vi "HFRR ADV v10.vi"() -> ()   [LabVIEW 2025] (continued)
            }
            "Rt 3" <- TRUE ("Rt 3")
          }
        }
        n2649 = case shown="True" w3152 {
          tunnel: [FALSE ("RUN") TRUE ("RUN")] -> w3151
          tunnel: [_ 2] -> w3145
          frame False {
          }
          frame True {
          }
        }
        n2650 = case shown="True" w3150 {
          tunnel: [FALSE ("RUN") TRUE ("RUN")] -> w3149
          tunnel: [_ 3] -> w3144
          frame False {
          }
          frame True {
          }
        }
        n2651 = case shown="\"Acquire\"" w3130 {
          tunnel: w3132 -> [_ w3363]
          frame Default {
            w3362 = 0.0 ("output")
            n2652 = local write "PID-out"(w3362) -> ()
            n2653 = local write "Frequency ( Hz )"(w3362) -> ()
          }
          frame "Acquire" {
            n2654 = stacked-sequence {
              frame #0 {
                n2655 = local read "Auto Start Test"() -> (w3365:bool)
                n2656 = case shown="True" w3365 {
                  tunnel: "RUN" -> [w3386 w3389]
                  tunnel: [w3386 w3388] -> w3366
                  frame False {
                  }
                  frame True {
                    n2657 = local read "Auto Start Temp"() -> (w3387:bool)
                    n2658 = Or(x=w3389, y=w3387) -> (x .or. y?=w3388:bool)
                  }
                }
                n2659 = local read "clk"() -> (w3385:dbl)
                n2660 = local read "Save"() -> (w3381:bool)
                n2661 = Equal?(x=w3385, y=0.0) -> (x = y?=w3382:bool)
                n2662 = And(x=w3382, y=w3381) -> (x .and. y?=w3383:bool)
                n2663 = Not(x="Engage") -> (.not. x?=w3372:bool)
                n2664 = case shown="True" w3366 {
                  tunnel: [w3397 w3415] -> w3368
                  frame False {
                    w3397 = 0.0
                    n2665 = local read "Auto Start Test"() -> (w3393:bool)
                    n2666 = local write "Reinit PID"(TRUE) -> ()
                    n2667 = local write "Start Time"(TRUE ("Start Time")) -> ()
                    n2668 = property on="Stroke" class="DigNum (strict)"("Visible"=TRUE) -> ()  [unwired: 2 in, 2 out]
                    n2669 = property on="Stroke 2" class="DigNum (strict)"("Visible"=FALSE) -> ()  [unwired: 2 in, 2 out]
                    n2670 = case shown="False" w3393 {
                      frame False {
                        n2671 = property on="Heater Button" class="Bool (strict)"("DisabledEnum"=T16."Enabled" ("Disabled")) -> ()  [unwired: 2 in, 2 out]
                        n2672 = property on="Humidity" class="Bool (strict)"("DisabledEnum"=T16."Enabled" ("Disabled")) -> ()  [unwired: 2 in, 2 out]
                      }
                      frame True {
                      }
                    }
                    n2673 = case shown="False" "TestCompFlg" {
                      frame False {
                        n2674 = local read "StartFlg"() -> (w3403:bool)
                        n2675 = case shown="True" w3403 {
                          frame False {
                          }
                          frame True {
                            n2676 = flat-sequence {
                              frame #0 {
                                n2677 = local read "EVENT LOG"() -> (w3405:string)
                                n2678 = call "Event Log.vi"("Content"="Test was interrupted", "EVENT LOG"=w3405) -> ("EVENT LOG"=w3406:string)  [unwired: 8 in, 1 out]
                                n2679 = local write "EVENT LOG"(w3406) -> ()
                              }
                              frame #1 {
                                w3407 = FALSE ("StartFlg")
                                n2680 = local write "Heater Button"(w3407) -> ()
                                n2681 = local write "StartFlg"(w3407) -> ()
                                n2682 = local write "Humidity"(w3407) -> ()
                              }
                            }
                          }
                        }
                      }
                      frame True {
                      }
                    }
                    n2683 = local write "String 14"("Test will autostart once parameters reach the set value." ("String 14")) -> ()
                    n2684 = local write "Old Pid Val"(w3397) -> ()
                  }
                  frame True {
                    n2685 = property on="Stroke 2" class="DigNum (strict)"("Visible"=TRUE) -> ()  [unwired: 2 in, 2 out]
                    n2686 = property on="Stroke" class="DigNum (strict)"("Visible"=FALSE) -> ()  [unwired: 2 in, 2 out]
                    n2687 = property on="STOP 2" class="Bool (strict)"("Disabled"=u8 2) -> ()  [unwired: 2 in, 2 out]
                    n2688 = local write "String 14"(" Running....." ("String 14")) -> ()
                    n2689 = property on="Heater Button" class="Bool (strict)"("DisabledEnum"=T16."Disabled and Grayed Out" ("Disabled")) -> ()  [unwired: 2 in, 2 out]
                    n2690 = property on="Humidity" class="Bool (strict)"("DisabledEnum"=T16."Disabled and Grayed Out" ("Disabled")) -> ()  [unwired: 2 in, 2 out]
                    n2691 = local read "PID Ref"() -> (w3426:bool)
                    n2692 = case shown="True" w3426 {
                      tunnel: [w3432 w3448] -> w3425
                      frame False {
                        n2693 = local read "Old Pid Val"() -> (w3432:dbl)
                      }
                      frame True {
                        n2694 = local read "Set Hz"() -> (w3441:dbl)
                        n2695 = local read "Frequency"() -> (w3452:dbl)
                        n2696 = Add(x=w3441, y=10.0) -> (x+y=w3450:dbl)
                        n2697 = Add(x=w3441, y=-10.0 ("Offset")) -> (x+y=w3459:dbl)
                        n2698 = Add(x=w3441, y=-10.0) -> (x+y=w3451:dbl)
                        n2699 = In Range and Coerce(upper limit=w3450, x=w3452, lower limit=w3451) -> (coerced(x)=w3440:dbl)  [unwired: 1 out]
                        n2700 = Or(x="Reinit PID", y="Reinit PID") -> (x .or. y?=w3449:bool)
                        n2701 = Multiply(x=w3459, y=0.1 ("Gain")) -> (x*y=w3438:dbl)
                        n2702 = local read "Elapsed time"() -> (w3445:dbl)
                        n2703 = local read "SPEED OUT:"() -> (w3460:dbl)
                        n2704 = Add(x=w3438, y=1.5) -> (x+y=w3436:dbl)
                        n2705 = call-poly <vilib>:"PID.vi"("reinitialize? (F)"=w3449, "output range"=cluster{"output high":dbl, "output low":dbl} {"output high"=1.0, "output low"=-1.0}, "PID gains"=T13 {"proportional gain (Kc)"=0.0005, "integral time (Ti, min)"=0.001, "derivative time (Td, min)"=0.0} ("Motor PID"), "process variable"=w3440, "setpoint"=w3441) -> ("output"=w3439:dbl)  [unwired: 5 in, 1 out]
                        n2706 = Multiply(x=w3436, y=w3460) -> (x*y=w3435:dbl)
                        n2707 = Greater?(x=w3445, y=0.05) -> (0:w3444:bool)
                        n2708 = case shown="True" w3444 {
                          tunnel: w3439 -> [_ w3462]
                          tunnel: [0.0 ("output") w3462] -> w3442
                          frame False {
                          }
                          frame True {
                            n2709 = local write "Reinit PID"(FALSE ("Reinit PID")) -> ()
                          }
                        }
                        n2710 = Multiply(x=w3435, y=0.8) -> (x*y=w3434:dbl)
                        n2711 = Add(x=w3434, y=w3442) -> (x+y=w3447:dbl)
                        n2712 = flat-sequence {
                          tunnel: [w3465] -> w3448
                          tunnel: w3447 -> [w3465]
                          frame #0 {
                            n2713 = local write "PID Ref"(FALSE ("PID Ref")) -> ()
                          }
                        }
                      }
                    }
                    "Old Pid Val" <- w3425
                    n2714 = case shown="True" "Start Time" {
                      selector: "Start Time" -> [_ w3428]
                      frame False {
                      }
                      frame True {
                        n2715 = Not(x=w3428) -> (.not. x?=w3427:bool)
                        n2716 = local write "Start Time"(w3427) -> ()
                        n2717 = local read "EVENT LOG"() -> (w3429:string)
                        n2718 = call "Event Log.vi"("Content"="Test in progress", "EVENT LOG"=w3429) -> ("EVENT LOG"=w3431:string)  [unwired: 8 in, 1 out]
                        n2719 = local write "EVENT LOG"(w3431) -> ()
                      }
                    }
                    n2720 = local read "Set Hz"() -> (w3422:dbl)
                    n2721 = call <vilib>:"Uniform White Noise Waveform.vi"() -> ("signal out"=w3421:waveform(dbl))  [unwired: 10 in, 1 out]
                    n2722 = local read "Freq"() -> (w3414:dbl)
                    n2723 = Add(x=w3422, y=w3421) -> (x+y=w3420:waveform(dbl))
                    n2724 = Multiply(x=w3420, y=ext 0.1) -> (x*y=w3416:waveform(ext))
                    n2725 = Multiply(x=w3414, y=0.9) -> (x*y=w3417:dbl)
                    n2726 = Add(x=w3416, y=w3417) -> (x+y=w3415:waveform(ext))
                    "StartFlg" <- TRUE ("StartFlg")
                  }
                }
                n2727 = case shown="True" w3383 {
                  frame False {
                  }
                  frame True {
                    n2728 = local write "clk"(10.0 ("clk")) -> ()
                    n2729 = Get Date/Time In Seconds() -> (seconds since 1Jan1904=w3468:timestamp)
                    n2730 = To Double Precision Float(number=w3468) -> (double precision float=w3466:dbl)
                    n2731 = local write "acq timer"(w3466) -> ()
                    n2732 = local write "act save time"(w3466) -> ()
                  }
                }
                n2733 = call "Elapsed Time"("Time Target (s)"="Countdown", "Reset"=w3372) -> ("Elapsed Time (s)"=w3377:dbl, "Time has Elapsed"=w3375:bool)  [unwired: 10 in, 6 out]
                "Countdown 2" <- w3377
                n2734 = Subtract(x=w3377, y=2.0) -> (x-y=w3380:dbl)
                n2735 = Less?(x=w3380, y="Countdown") -> (x < y?=w3378:bool)
                n2736 = And(x=w3378, y=w3375) -> (x .and. y?=w3374:bool)
                n2737 = case shown="True" w3374 {
                  frame False {
                  }
                  frame True {
                    (unwired) dbl[] [] ("History Data")
                    n2738 = local write "Engage"(FALSE ("Engage")) -> ()
                    n2739 = local write "RUN"(TRUE ("RUN")) -> ()
                    n2740 = local read "Humidity ( %RH )"() -> (→"Rh Before":dbl)
                  }
                }
                n2741 = local read "Test \nStatus"() -> (w3370:bool)
                n2742 = Select(t=w3368, s=w3370, f=0.0) -> (s? t:f=w3369:dbl)
                n2743 = local write "Frequency ( Hz )"(w3369) -> ()
                n2744 = local write "Freq"(w3369) -> ()
              }
              frame #1 {
                w3491 = 1000000.0 ("x")
                # "Elapsed time\ncof\nstroke\nAir temp\nTemp\nHumidity"
                # "acq timer\n\nact save time"
                # "convert to microseconds"
                n2745 = local read "COUNT"() -> (w3474:i32)
                n2746 = local read "Rate"() -> (w3487:dbl)
                n2747 = Divide(x=w3491, y=w3487) -> (x/y=w3492:dbl)
                n2748 = Greater Or Equal?(x=w3474, y=250) -> (x >= y?=w3473:bool)
                n2749 = Get Date/Time In Seconds() -> (seconds since 1Jan1904=w3494:timestamp)
                n2750 = case shown="True" w3473 {
                  frame False {
                    n2751 = local read "COUNT"() -> (w3495:i32)
                    n2752 = Increment(x=w3495) -> (x+1=w3496:i32)
                    n2753 = local write "COUNT"(w3496) -> ()
                  }
                  frame True {
                    n2754 = local write "COUNT"(0 ("COUNT")) -> ()
                  }
                }
                n2755 = local read "Samplingtime 2"() -> (w3472:dbl)
                n2756 = local read "act save time"() -> (w3489:dbl)
                n2757 = Divide(x=w3492, y=w3491) -> (x/y=w3490:dbl)
                n2758 = To Double Precision Float(number=w3494) -> (double precision float=w3483:dbl)
                n2759 = Add(x=w3489, y=w3472) -> (x+y=w3488:dbl)
                n2760 = local read "acq timer"() -> (w3493:dbl)
                n2761 = local read "COUNT"() -> (w3476:i32)
                n2762 = Greater Or Equal?(x=w3483, y=w3488) -> (x >= y?=w3471:bool)
                n2763 = Multiply(x=w3490, y=w3476) -> (x*y=w3482:dbl)
                n2764 = Subtract(x=w3483, y=w3493) -> (x-y=w3485:dbl)
                n2765 = local read "Save"() -> (w3486:bool)
                n2766 = Add(x=w3485, y=w3482) -> (x+y=w3469:dbl)
                "Elapsed time 3" <- w3469
                n2767 = And(x=w3471, y=w3486) -> (x .and. y?=w3484:bool)
                n2768 = Divide(x=w3469, y=60.0) -> (x/y=w3480:dbl)
                n2769 = local read "Test \nStatus"() -> (w3470:bool)
                n2770 = local read "clk"() -> (w3477:dbl)
                n2771 = Equal?(x=w3477, y=10.0) -> (x = y?=w3479:bool)
                n2772 = case shown="True" w3484 {
                  tunnel: w3483 -> [_ w3598]
                  tunnel: [FALSE ("Boolean 2") TRUE ("Boolean 2")] -> _
                  frame False {
                  }
                  frame True {
                    w3545 = ";" ("Substring")
                    # "Pid out/\nFreq response value"
                    n2773 = local write "act save time"(w3598) -> ()
                    n2774 = local read "FILE"() -> (w3539:string)
                    n2775 = call "file check.vi"("file name in"=w3539) -> ("error out"=w3542:errorcluster, "file name out"=w3537:string)  [unwired: 9 in]
                    n2776 = call "FILE PATH CREATION.vi"("error in"=w3542, "FILE NAME :"=w3537) -> ("FILE OUT"=w3540:path)  [unwired: 8 in, 1 out]
                    n2777 = Concatenate Strings(w3537, ".dgf" ("Substring")) -> (w3541:string)
                    n2778 = local read "Set Strk"() -> (w3569:dbl)
                    n2779 = local read "Stroke"() -> (w3560:dbl)
                    n2780 = local read "FF 2"() -> (→"Frictional Force ( N )" →"Frictional Force ( N )":dbl)
                    n2781 = Build Path(base path=w3540, name or relative path=w3541) -> (appended path=w3536:path)
                    n2782 = Subtract(x=w3560, y=w3569) -> (x-y=w3566:dbl)
                    n2783 = local read "COF 2"() -> (w3551:dbl)
                    "cof" <- w3551
                    "Coefficient of Friction" <- w3551
                    "COF 4" <- w3551
                    "Coefficient of Friction" <- w3551
                    n2784 = Multiply(x=w3566, y=0.05) -> (x*y=w3568:dbl)
                    n2785 = local read "TEMP"() -> (w3555:dbl)
                    "Temp" <- w3555
                    "Temperature ( Deg C )" <- w3555
                    n2786 = Add(x=w3568, y=w3569) -> (x+y=w3549:dbl)
                    "Stroke Ln" <- w3549
                    "Disp" <- w3549
                    n2787 = local read "ecr"() -> (w3552:dbl)
                    "Electrical Contact Resistance ( % )" <- w3552
                    n2788 = local read "Humidity ( %RH )"() -> (w3554:dbl)
                    "Humidity ( %RH )" <- w3554
                    "Humidity ( %RH )" <- w3554
                    n2789 = local read "Frequency ( Hz )"() -> (w3562:dbl)
                    n2790 = local read "Elapsed time"() -> (w3591:dbl)
                    n2791 = disable-structure shown="Disabled" {
                      frame Disabled {
                        n2792 = local read "ecr 3"() -> ()  [unwired: 1 in]
                      }
                      frame Enabled {
                      }
                    }
                    n2793 = local read "AIR TEMP"() -> (w3559:dbl)
                    n2794 = local read "PID-out"() -> (w3565:dbl)
                    n2795 = local write "Temperature ( Deg C )"(w3555) -> ()
                    n2796 = Number To Fractional String(number=w3549, width (-)=i16 9 ("precision (6)"), precision (6)=i16 6) -> (F-format string=w3584:string)  [unwired: 1 in]
                    n2797 = Number To Fractional String(number=w3559, width (-)=i16 9 ("precision (6)"), precision (6)=i16 3) -> (F-format string=w3583:string)  [unwired: 1 in]
                    n2798 = Number To Fractional String(number=w3555, width (-)=i16 9 ("precision (6)"), precision (6)=i16 3) -> (F-format string=w3580:string)  [unwired: 1 in]
                    n2799 = Number To Fractional String(number=w3554, width (-)=i16 9 ("precision (6)"), precision (6)=i16 3) -> (F-format string=w3577:string)  [unwired: 1 in]
                    n2800 = Number To Fractional String(number=w3552, width (-)=i16 9 ("precision (6)"), precision (6)=i16 3) -> (F-format string=w3574:string)  [unwired: 1 in]
                    n2801 = Number To Fractional String(number=w3565, width (-)=i16 9 ("precision (6)"), precision (6)=i16 3) -> (F-format string=w3570:string)  [unwired: 1 in]
                    n2802 = Number To Fractional String(number=w3562, width (-)=i16 9 ("precision (6)"), precision (6)=i16 3) -> (F-format string=w3561:string)  [unwired: 1 in]
                    n2803 = Number To Fractional String(number=w3551, width (-)=i16 9 ("precision (6)"), precision (6)=i16 6) -> (F-format string=w3592:string)  [unwired: 1 in]
                    n2804 = Number To Fractional String(number=w3591, width (-)=i16 14 ("precision (6)"), precision (6)=i16 3) -> (F-format string=w3593:string)  [unwired: 1 in]
                    n2805 = Bundle("y"=1.02, w3549, "y"=0.98) -> (w3553:cluster{"y":dbl, dbl, "y":dbl})  [unwired: 1 in]
                    n2806 = Number To Fractional String(number="Ambient Humidity :", width (-)=i16 9 ("precision (6)"), precision (6)=i16 6) -> (F-format string=w3543:string)  [unwired: 1 in]
                    n2807 = local read "RUN"() -> (w3550:bool)
                    n2808 = case shown="True" w3550 {
                      tunnel: w3553 -> [_ w3603]
                      tunnel: w3549 -> [_ w3602]
                      tunnel: w3549 -> [_ w3601]
                      tunnel: w3549 -> [_ w3600]
                      frame False {
                      }
                      frame True {
                        "Stroke ( mm )" <- w3603
                        "Stroke ( mm )" <- w3603
                        "Stroke 4" <- w3602
                        "Stroke 3" <- w3601
                        "Stroke 2" <- w3600
                      }
                    }
                    n2809 = Concatenate Strings(w3593, w3545, w3592, w3545, w3584, w3545, w3583, w3545, w3580, w3545, w3577, w3545, w3574, w3545, w3570, w3545, w3561, w3545, w3543, "\r") -> (w3590:string)
                    n2810 = call <vilib>:"Write Characters To File.vi"("append to file? (new file:F)"=TRUE, "character string"=w3590, "file path (dialog if empty)"=w3536) -> ()  [unwired: 2 in, 1 out]
                    "refresh flag" <- TRUE ("refresh flag")
                  }
                }
                n2811 = case shown="True" w3470 {
                  tunnel: w3480 -> [_ w3506]
                  tunnel: w3485 -> [_ w3516]
                  tunnel: [0.0 w3512] -> _
                  tunnel: w3479 -> [_ w3511]
                  tunnel: [0.0 w3510] -> _
                  tunnel: w3469 -> [_ w3510]
                  tunnel: w3483 -> [w3499 _]
                  frame False {
                    n2812 = local write "acq timer"(w3499) -> ()
                    n2813 = local write "Test Duration Status"(0.0 ("Test Duration Status")) -> ()
                  }
                  frame True {
                    n2814 = local read "Set Hz"() -> (w3513:dbl)
                    n2815 = local write "Elapsed time"(w3506) -> ()
                    n2816 = local read "test time"() -> (w3505:dbl)
                    n2817 = Multiply(x=w3516, y=w3513) -> (x*y=w3515:dbl)
                    n2818 = case shown="False" w3511 {
                      tunnel: w3515 -> [w3517 _]
                      tunnel: [w3517 1.0] -> w3512
                      frame False {
                        n2819 = local write "Cycles elapsed"(w3517) -> ()
                      }
                      frame True {
                      }
                    }
                    n2820 = Greater?(x=w3506, y=w3505) -> (0:w3514:bool)
                    n2821 = Subtract(x=w3505, y=w3506) -> (x-y=w3504:dbl)
                    "time" <- w3504
                    n2822 = Multiply(x=w3504, y=60.0) -> (x*y=w3503:dbl)
                    n2823 = local write "Time Remaining"(w3503) -> ()
                    n2824 = local write "Remaining Time"(w3503) -> ()
                    n2825 = case shown="True" w3514 {
                      frame False {
                      }
                      frame True {
                        w3519 = T16."Enabled" ("Disabled")
                        w3523 = "" ("FILE")
                        w3524 = TRUE ("Visible")
                        n2826 = local write "Humidity"(FALSE ("Humidity")) -> ()
                        n2827 = local write "RUN"(FALSE ("OK Button 2")) -> ()
                        n2828 = local write "Heater Button"(FALSE ("Heater Button")) -> ()
                        n2829 = local write "Auto Start Test"(FALSE ("Auto Start Test")) -> ()
                        n2830 = local write "TestCompFlg"(TRUE ("StpFlg")) -> ()
                        n2831 = local read "Humidity ( %RH )"() -> (→"Rh After":dbl)
                        n2832 = property on="STOP 2" class="Bool (strict)"("Disabled"=u8 0) -> ()  [unwired: 2 in, 2 out]
                        n2833 = local read "EVENT LOG"() -> (w3529:string)
                        n2834 = call "Event Log.vi"("Content"="Test Completed", "EVENT LOG"=w3529) -> ("EVENT LOG"=w3528:string)  [unwired: 8 in, 1 out]
                        n2835 = property on="RUN" class="Bool (strict)"("Visible"=w3524) -> ()  [unwired: 2 in, 2 out]
                        n2836 = property on="Auto Start Test" class="Bool (strict)"("Visible"=w3524) -> ()  [unwired: 2 in, 2 out]
                        n2837 = local write "Batch Ref Num :"(w3523) -> ()
                        n2838 = local write "FILE"(w3523) -> ()
                        n2839 = local write "EVENT LOG"(w3528) -> ()
                        n2840 = local write "TEST FILE NAM,E SAVED"(FALSE ("TEST FILE NAM,E SAVED")) -> ()
                        n2841 = local write "Fuel Discription :"(w3523) -> ()
                        n2842 = local write "Remarks :"(w3523) -> ()
                        n2843 = local write "Main Dashboard Buttons"(T1."Imaging" ("Main Dashboard Buttons")) -> ()
                        n2844 = local write "Main Tab"(T2."Adv Scar" ("Main Tab")) -> ()
                        n2845 = property on="FRICVALZ 2" class="Bool (strict)"("DisabledEnum"=w3519) -> ()  [unwired: 2 in, 2 out]
                        n2846 = property on="FRICVALZ 3" class="Bool (strict)"("DisabledEnum"=w3519) -> ()  [unwired: 2 in, 2 out]
                        n2847 = property on="FRICVALZ 4" class="Bool (strict)"("DisabledEnum"=w3519) -> ()  [unwired: 2 in, 2 out]
                      }
                    }
                    n2848 = Divide(x=w3506, y=w3505) -> (x/y=w3509:dbl)
                    n2849 = Multiply(x=w3509, y=100.0) -> (x*y=w3507:dbl)
                    n2850 = local write "Test Duration Status"(w3507) -> ()
                  }
                }
              }
              frame #2 {
                n2851 = case shown="True" "Heater Button" {
                  tunnel: [0.0 ("output") w3627] -> w3604
                  frame False {
                    w3607 = TRUE ("tmpchk")
                    n2852 = local read "TEMP"() -> (w3608:dbl)
                    n2853 = local write "Temp ini"(w3608) -> ()
                    n2854 = local write "Reset 4"(w3607) -> ()
                    n2855 = local write "tmpchk"(w3607) -> ()
                    n2856 = local write "reinit"(TRUE ("reinit")) -> ()
                    n2857 = local write "manual temp log"(TRUE ("manual temp log")) -> ()
                  }
                  frame True {
                    # "Logic to turn off\nthe heater when \ntemp is not rising.\nTime - 60 sec\nDelta t- 5°c"
                    n2858 = local read "Temp ini"() -> (w3615:dbl)
                    n2859 = local read "Auto Start Test"() -> (w3611:bool)
                    n2860 = Less?(x=w3615, y=53.0) -> (x < y?=w3613:bool)
                    n2861 = case shown="False" w3611 {
                      frame False {
                        n2862 = local read "Set Temp"() -> (w3638:dbl)
                        n2863 = local read "TEMP"() -> (w3637:dbl)
                        n2864 = Subtract(x=w3638, y=w3637) -> (x-y=w3636:dbl)
                        n2865 = Absolute Value(x=w3636) -> (abs(x)=w3635:dbl)
                        n2866 = Less?(x=w3635, y=0.5) -> (x < y?=w3633:bool)
                        n2867 = case shown="True" w3633 {
                          tunnel: "manual temp log" -> [_ w3639]
                          frame False {
                          }
                          frame True {
                            n2868 = case shown="True" w3639 {
                              selector: w3639 -> [_ w3640]
                              frame False {
                              }
                              frame True {
                                # "#Event log"
                                n2869 = Not(x=w3640) -> (.not. x?=w3641:bool)
                                n2870 = local write "manual temp log"(w3641) -> ()
                                n2871 = local read "EVENT LOG"() -> (w3644:string)
                                n2872 = call "Event Log.vi"("Content"="Target Temperature reached", "EVENT LOG"=w3644) -> ("EVENT LOG"=w3643:string)  [unwired: 8 in, 1 out]
                                n2873 = local write "EVENT LOG"(w3643) -> ()
                              }
                            }
                          }
                        }
                      }
                      frame True {
                        n2874 = local write "manual temp log"(TRUE ("manual temp log")) -> ()
                      }
                    }
                    n2875 = And(x="tmpchk", y=w3613) -> (x .and. y?=w3616:bool)
                    n2876 = case shown="True" w3616 {
                      frame False {
                      }
                      frame True {
                        n2877 = call "Elapsed Time8"("Time Target (s)"=300.0, "Reset"="Reset 4") -> ("Time has Elapsed"=w3646:bool)  [unwired: 10 in, 7 out]
                        n2878 = flat-sequence {
                          tunnel: w3646 -> [_]
                          frame #0 {
                            n2879 = local write "Reset 4"(FALSE ("Reset 4")) -> ()
                          }
                        }
                        n2880 = case shown="True" w3646 {
                          frame False {
                          }
                          frame True {
                            n2881 = local read "Temp ini"() -> (w3653:dbl)
                            n2882 = Add(x=w3653, y=5.0) -> (x+y=w3651:dbl)
                            n2883 = local read "TEMP"() -> (w3654:dbl)
                            n2884 = Greater?(x=w3654, y=w3651) -> (0:w3652:bool)
                            n2885 = case shown="False" w3652 {
                              frame False {
                                n2886 = local write "Heater Button"(FALSE ("Heater Button")) -> ()
                              }
                              frame True {
                                n2887 = local write "tmpchk"(FALSE ("tmpchk")) -> ()
                              }
                            }
                          }
                        }
                      }
                    }
                    n2888 = local read "Set Temp"() -> (w3624:dbl)
                    n2889 = local read "TEMP"() -> (w3618:dbl)
                    n2890 = call-poly <vilib>:"PID.vi"("reinitialize? (F)"="reinit", "output range"="output range", "dt (s)"=-1.0, "PID gains"="Temp PID gains", "process variable"=w3618, "setpoint"=w3624) -> ("output"=w3621:dbl)  [unwired: 4 in, 1 out]
                    n2891 = Subtract(x=w3624, y=w3618) -> (x-y=w3626:dbl)
                    n2892 = Add(x=w3624, y=0.5) -> (x+y=w3622:dbl)
                    n2893 = Greater Or Equal?(x=w3618, y=w3622) -> ()  [unwired: 1 out]
                    n2894 = Select(t=0.0, s=FALSE, f=w3621) -> (s? t:f=w3620:dbl)
                    "PID output" <- w3620
                    n2895 = flat-sequence {
                      tunnel: w3620 -> [w3657]
                      tunnel: [w3657] -> w3627
                      frame #0 {
                        n2896 = local write "reinit"(FALSE ("reinit")) -> ()
                      }
                    }
                    n2897 = Bundle(w3626, "output"=w3620, "TEMP"=w3618) -> (→"gTEMP 3":cluster{dbl, "output":dbl, "TEMP":dbl})  [unwired: 1 in]
                  }
                }
                "PID-out" <- w3604
              }
              frame #3 {
                n2898 = local read "TEMP"() -> (w3659:dbl)
                n2899 = Greater Or Equal?(x=w3659, y="Set Temp 2") -> (x >= y?=w3664:bool)
                n2900 = case shown="True" w3664 {
                  tunnel: [FALSE TRUE] -> w3662
                  frame False {
                  }
                  frame True {
                  }
                }
                "Status 13" <- w3662
                n2901 = And(x=w3662, y="trip1 8") -> (x .and. y?=w3661:bool)
                n2902 = case shown="True" w3661 {
                  frame False {
                    n2903 = local write "Heater Trip Temp"(TRUE ("Heater Trip Temp")) -> ()
                  }
                  frame True {
                    w3667 = FALSE ("OK Button 2")
                    n2904 = case shown="True" "Heater Trip Temp" {
                      selector: "Heater Trip Temp" -> [_ w3669]
                      frame False {
                      }
                      frame True {
                        n2905 = Not(x=w3669) -> (.not. x?=w3668:bool)
                        n2906 = local read "EVENT LOG"() -> (w3672:string)
                        n2907 = local write "Heater Trip Temp"(w3668) -> ()
                        n2908 = call "Event Log.vi"("Content"="Heater Trip", "EVENT LOG"=w3672) -> ("EVENT LOG"=w3671:string)  [unwired: 8 in, 1 out]
                        n2909 = local write "EVENT LOG"(w3671) -> ()
                      }
                    }
                    n2910 = local write "RUN"(w3667) -> ()
                    n2911 = property on="Auto Start Test" class="Bool (strict)"("Value"=w3667) -> ()  [unwired: 2 in, 2 out]
                    n2912 = local write "Heater Button"(w3667) -> ()
                  }
                }
              }
            }
            n2913 = case shown="False" w3363 {
              frame False {
                n2914 = disable-structure shown="Enabled" {
                  frame Enabled {
                    n2915 = stacked-sequence {
                      frame #0 {
                        n2916 = local write "RUN"(FALSE ("OK Button 2")) -> ()
                      }
                      frame #1 {
                      }
                    }
                  }
                  frame Disabled {
                  }
                }
              }
              frame True {
              }
            }
          }
        }
        n2917 = local read "airtempflg"() -> (w3155:bool)
        n2918 = Or(x=w3155, y=w3153) -> (x .or. y?=w3156:bool)
        n2919 = Insert Into Array(array=string[] ["Air Temperature has reached set value,", "Humidity has reached set value,", "Sample Temperaturehas reached set value,", ""], index=0, new element="") -> (w3141:string[])
        n2920 = Build Array(w3146, w3145, w3144) -> (w3142:i32[])
        n2921 = disable-structure shown="Disabled" {
          disable-tunnel: w3156 -> [w3233 _]
          disable-tunnel: w3151 -> [w3232 _]
          disable-tunnel: w3149 -> [w3231 _]
          frame Disabled {
            n2922 = Compound Arithmetic op=AND(w3233, w3232, w3231) -> ()  [unwired: 1 out]
            n2923 = case shown="True" {
              selector: _ -> [_ _]
              frame False {
              }
              frame True {
                w3234 = FALSE ("autostrtflg")
                n2924 = local write "RUN"(TRUE ("RUN")) -> ()
                n2925 = local write "autostrtflg"(w3234) -> ()
                n2926 = local write "autostart"(w3234) -> ()
                n2927 = local write "String 14"(" Running....." ("String 14")) -> ()
              }
            }
          }
          frame Enabled {
          }
        }
        n2928 = for {
          tunnel: w3142 -> [w3284] mode=indexing
          tunnel: w3141 -> [w3283]
          shift-right: [w3280] -> w3140
          shift-left: "" -> [w3282]
          n2929 = Index Array(array=w3283, index=w3284) -> (element=w3281:string)
          n2930 = Concatenate Strings(w3281, w3282) -> (w3280:string)
        }
        n2931 = local write "autostart 2"(w3140) -> ()
        n2932 = local read "Reset Graph"() -> (w3129:bool)
        n2933 = case shown="True" w3129 {
          selector: w3129 -> [_ w3183]
          frame False {
          }
          frame True {
            w3197 = 0.0 ("X Scale.Range:Maximum")
            n2934 = Not(x=w3183) -> (.not. x?=w3182:bool)
            n2935 = local write "Reset Graph"(w3182) -> ()
            n2936 = property on="Electrical Contact Resistance ( % )" class="WFChart (strict)"("XScale.Maximum"=600.0 ("X Scale.Range:Maximum"), "XScale.Minimum"=0.0 ("X Scale.Range:Minimum"), "YScale.Maximum"=100.0 ("Y Scale.Range:Maximum"), "YScale.Minimum"=0.0 ("Y Scale.Range:Minimum")) -> ()  [unwired: 2 in, 2 out]
            n2937 = property on="Frictional Force ( N )" class="WFChart (strict)"("XScale.Maximum"=600.0 ("X Scale.Range:Maximum"), "XScale.Minimum"=0.0 ("X Scale.Range:Minimum"), "YScale.Maximum"=100.0 ("Y Scale.Range:Maximum"), "YScale.Minimum"=0.0 ("Y Scale.Range:Minimum")) -> ()  [unwired: 2 in, 2 out]
            n2938 = property on="Temperature ( Deg C )" class="WFChart (strict)"("XScale.Maximum"=600.0 ("X Scale.Range:Maximum"), "XScale.Minimum"=0.0 ("X Scale.Range:Minimum"), "YScale.Maximum"=100.0 ("Y Scale.Range:Maximum"), "YScale.Minimum"=0.0 ("Y Scale.Range:Minimum")) -> ()  [unwired: 2 in, 2 out]
            n2939 = property on="Humidity ( %RH )" class="WFChart (strict)"("XScale.Maximum"=600.0 ("X Scale.Range:Maximum"), "XScale.Minimum"=0.0 ("X Scale.Range:Minimum"), "YScale.Maximum"=100.0 ("Y Scale.Range:Maximum"), "YScale.Minimum"=0.0 ("Y Scale.Range:Minimum")) -> ()  [unwired: 2 in, 2 out]
            n2940 = property on="Stroke ( mm )" class="WFChart (strict)"("XScale.Maximum"=600.0 ("X Scale.Range:Maximum"), "XScale.Minimum"=0.0 ("X Scale.Range:Minimum"), "YScale.Maximum"=100.0 ("Y Scale.Range:Maximum"), "YScale.Minimum"=0.0 ("Y Scale.Range:Minimum")) -> ()  [unwired: 2 in, 2 out]
            n2941 = property on="Coefficient of Friction" class="WFChart (strict)"("XScale.Maximum"=600.0 ("X Scale.Range:Maximum"), "XScale.Minimum"=0.0 ("X Scale.Range:Minimum"), "YScale.Maximum"=100.0 ("Y Scale.Range:Maximum"), "YScale.Minimum"=0.0 ("Y Scale.Range:Minimum")) -> ()  [unwired: 2 in, 2 out]
            n2942 = property on="Electrical Contact Resistance ( % )" class="WFChart (strict)"("XScale.Minimum"=0.0 ("X Scale.Range:Minimum"), "XScale.Maximum"=600.0 ("X Scale.Range:Maximum"), "YScale.Minimum"=0.0 ("Y Scale.Range:Minimum"), "YScale.Maximum"=100.0 ("Y Scale.Range:Maximum")) -> ()  [unwired: 2 in, 2 out]
            n2943 = property on="Temperature ( Deg C )" class="WFChart (strict)"("XScale.Minimum"=0.0 ("X Scale.Range:Minimum"), "XScale.Maximum"=600.0 ("X Scale.Range:Maximum"), "YScale.Minimum"=0.0 ("Y Scale.Range:Minimum"), "YScale.Maximum"=100.0 ("Y Scale.Range:Maximum")) -> ()  [unwired: 2 in, 2 out]
            n2944 = property on="Coefficient of Friction" class="WFChart (strict)"("XScale.Minimum"=0.0 ("X Scale.Range:Minimum"), "XScale.Maximum"=600.0 ("X Scale.Range:Maximum"), "YScale.Maximum"=1.0 ("X Scale.Range:Minimum"), "YScale.Minimum"=0.0 ("X Scale.Range:Minimum")) -> ()  [unwired: 2 in, 2 out]
            n2945 = property on="Frictional Force ( N )" class="WFChart (strict)"("XScale.Maximum"=600.0 ("X Scale.Range:Maximum"), "XScale.Minimum"=w3197, "YScale.Maximum"=10.0 ("Y Scale.Range:Maximum"), "YScale.Minimum"=w3197) -> ()  [unwired: 2 in, 2 out]
            n2946 = property on="Stroke ( mm )" class="WFChart (strict)"("XScale.Maximum"=600.0 ("X Scale.Range:Maximum"), "XScale.Minimum"=0.0 ("X Scale.Range:Minimum"), "YScale.Maximum"=100.0 ("Y Scale.Range:Maximum"), "YScale.Minimum"=0.0 ("Y Scale.Range:Minimum")) -> ()  [unwired: 2 in, 2 out]
            n2947 = property on="Humidity ( %RH )" class="WFChart (strict)"("XScale.Maximum"=600.0 ("X Scale.Range:Maximum"), "XScale.Minimum"=0.0 ("X Scale.Range:Minimum"), "YScale.Maximum"=100.0 ("Y Scale.Range:Maximum"), "YScale.Minimum"=0.0 ("Y Scale.Range:Minimum")) -> ()  [unwired: 2 in, 2 out]
          }
        }
      }
      frame "Compare Files" {
        # "Elapsed time\ncof\nstroke\nAir temp\nTemp\nHumidity"
        n2948 = case shown="True" "RSTV1 2" {
          frame False {
          }
          frame True {
            n2949 = property on="Humidity ( %RH )" class="XYGraph (strict)"("Y Scale.Display Format:Precision"=u8 0 ("Y Scale.Format & Precision:Precision")) -> ()  [unwired: 2 in, 2 out]
            n2950 = property on="Humidity ( %RH )" class="XYGraph (strict)"("X Scale.Range:Minimum"=0.0, "X Scale.Range:Maximum"=75.0, "Y Scale.Range:Minimum"=48.0, "Y Scale.Range:Maximum"=58.0) -> ()  [unwired: 2 in, 2 out]
          }
        }
        n2951 = case shown="True" "RST CP 2" {
          frame False {
          }
          frame True {
            n2952 = property on="XY Graph 13" class="XYGraph (strict)"("Y Scale.Display Format:Precision"=u8 0 ("Y Scale.Format & Precision:Precision")) -> ()  [unwired: 2 in, 2 out]
            n2953 = property on="XY Graph 13" class="XYGraph (strict)"("X Scale.Range:Minimum"=0.0, "X Scale.Range:Maximum"=75.0, "Y Scale.Range:Minimum"=0.0, "Y Scale.Range:Maximum"=100.0) -> ()  [unwired: 2 in, 2 out]
          }
        }
        n2954 = case shown="True" "RST CP" {
          frame False {
          }
          frame True {
            n2955 = property on="Sample Temperature ( °C )" class="XYGraph (strict)"("Y Scale.Display Format:Precision"=u8 2 ("Y Scale.Format & Precision:Precision")) -> ()  [unwired: 2 in, 2 out]
            n2956 = property on="Sample Temperature ( °C )" class="XYGraph (strict)"("X Scale.Range:Minimum"=0.0, "X Scale.Range:Maximum"=75.0, "Y Scale.Range:Minimum"=58.0, "Y Scale.Range:Maximum"=62.0) -> ()  [unwired: 2 in, 2 out]
          }
        }
        n2957 = case shown="True" "RSTV1 3" {
          frame False {
          }
          frame True {
            n2958 = property on="Air Temperature  ( °C )" class="XYGraph (strict)"("Y Scale.Display Format:Precision"=u8 2 ("Y Scale.Format & Precision:Precision")) -> ()  [unwired: 2 in, 2 out]
            n2959 = property on="Air Temperature  ( °C )" class="XYGraph (strict)"("X Scale.Range:Minimum"=0.0 ("Y Scale.Range:Minimum"), "X Scale.Range:Maximum"=75.0 ("Y Scale.Range:Maximum"), "Y Scale.Range:Minimum"=20.0 ("X Scale.Range:Minimum"), "Y Scale.Range:Maximum"=26.0 ("X Scale.Range:Maximum")) -> ()  [unwired: 2 in, 2 out]
          }
        }
        n2960 = case shown="True" "RSTV1 4" {
          frame False {
          }
          frame True {
            n2961 = property on="Stroke ( mm )" class="XYGraph (strict)"("Y Scale.Display Format:Precision"=u8 2 ("Y Scale.Format & Precision:Precision")) -> ()  [unwired: 2 in, 2 out]
            n2962 = property on="Stroke ( mm )" class="XYGraph (strict)"("X Scale.Range:Minimum"=0.0 ("Y Scale.Range:Maximum"), "X Scale.Range:Maximum"=75.0 ("X Scale.Range:Minimum"), "Y Scale.Range:Minimum"=0.98, "Y Scale.Range:Maximum"=1.02) -> ()  [unwired: 2 in, 2 out]
          }
        }
        n2963 = case shown="True" "rstv2" {
          frame False {
          }
          frame True {
            n2964 = property on="Coefficient Of Friction" class="XYGraph (strict)"("Y Scale.Display Format:Precision"=u8 3 ("Y Scale.Format & Precision:Precision")) -> ()  [unwired: 2 in, 2 out]
            n2965 = property on="Coefficient Of Friction" class="XYGraph (strict)"("X Scale.Range:Minimum"=0.0 ("Y Scale.Range:Maximum"), "X Scale.Range:Maximum"=75.0, "Y Scale.Range:Minimum"=0.0, "Y Scale.Range:Maximum"=1.0 ("X Scale.Range:Minimum")) -> ()  [unwired: 2 in, 2 out]
          }
        }
        n2966 = case shown="True" "RST CP 3" {
          frame False {
          }
          frame True {
            n2967 = property on="Air Temp ( °C ) vs Humidity ( % RH )" class="XYGraph (strict)"("X Scale.Range:Minimum"=18.0, "X Scale.Range:Maximum"=28.0 ("X Scale.Range:Minimum"), "Y Scale.Range:Minimum"=30.0 ("X Scale.Range:Minimum"), "Y Scale.Range:Maximum"=70.0 ("X Scale.Range:Minimum")) -> ()  [unwired: 2 in, 2 out]
          }
        }
        n2968 = case shown="True" "OPEN 1" {
          frame False {
          }
          frame True {
            (unwired) 0  # existing file
            w3948 = "Choose a datalog file to open"  # prompt
            n2969 = local write "OPEN 1"(FALSE ("OPEN 1")) -> ()
            n2970 = String To Path(string="C:\\LAB-IQ\\Data\\") -> (path=w3933:path)
            n2971 = File Dialog(6:"*.dgf" ("pattern"), 7:w3948, 11:w3933) -> (0:w3931:errorcluster, 3:w3939:path)  [unwired: 4 in, 2 out]
            n2972 = Unbundle(w3931) -> ()  [unwired: 3 out]
            n2973 = Strip Path(path=w3939) -> (name=w3938:string)  [unwired: 1 out]
            n2974 = Path To String(path=w3939) -> (string=w3934:string)
            "string1" <- w3934
            n2975 = Match Pattern(string=w3938, regular expression=".dgf") -> (before substring=→"String Control":string)  [unwired: 1 in, 3 out]
            n2976 = Match Pattern(string=w3934, regular expression=".dgf" ("substring (\"\")")) -> (before substring=w3944:string)  [unwired: 1 in, 3 out]
            n2977 = Concatenate Strings(w3944, ".duf" ("Substring")) -> (w3940:string)
            n2978 = String To Path(string=w3940) -> (path=w3945:path)
            n2979 = call <vilib>:"Read Characters From File.vi"("file path (dialog if empty)"=w3945, "start of read offset (chars.:0)"=60 ("start of read offset (chars.: 0)")) -> ("character string"=→"String Control 2":string)  [unwired: 4 in, 3 out]
          }
        }
        n2980 = case shown="True" "OPEN 2" {
          frame False {
          }
          frame True {
            (unwired) 0  # existing file
            w3966 = "Choose a datalog file to open"  # prompt
            n2981 = local write "OPEN 2"(FALSE ("OPEN 1")) -> ()
            n2982 = String To Path(string="C:\\LAB-IQ\\Data\\") -> (path=w3951:path)
            n2983 = File Dialog(6:"*.dgf" ("pattern"), 7:w3966, 11:w3951) -> (0:w3949:errorcluster, 3:w3957:path)  [unwired: 4 in, 2 out]
            n2984 = Unbundle(w3949) -> ()  [unwired: 3 out]
            n2985 = Strip Path(path=w3957) -> (name=w3955:string)  [unwired: 1 out]
            n2986 = Path To String(path=w3957) -> (string=w3952:string)
            "string1 2" <- w3952
            n2987 = Match Pattern(string=w3955, regular expression=".dgf") -> (before substring=→"String Control 3":string)  [unwired: 1 in, 3 out]
            n2988 = Match Pattern(string=w3952, regular expression=".dgf" ("substring (\"\")")) -> (before substring=w3963:string)  [unwired: 1 in, 3 out]
            n2989 = Concatenate Strings(w3963, ".duf" ("Substring")) -> (w3960:string)
            n2990 = String To Path(string=w3960) -> (path=w3958:path)
            n2991 = call <vilib>:"Read Characters From File.vi"("file path (dialog if empty)"=w3958, "start of read offset (chars.:0)"=60 ("start of read offset (chars.: 0)")) -> ("character string"=→"String Control 4":string)  [unwired: 4 in, 3 out]
          }
        }
        n2992 = case shown="True" "OPEN 3" {
          frame False {
          }
          frame True {
            (unwired) 0  # existing file
            w3984 = "Choose a datalog file to open"  # prompt
            n2993 = local write "OPEN 3"(FALSE ("OPEN 1")) -> ()
            n2994 = String To Path(string="C:\\LAB-IQ\\Data\\") -> (path=w3969:path)
            n2995 = File Dialog(6:"*.dgf" ("pattern"), 7:w3984, 11:w3969) -> (0:w3967:errorcluster, 3:w3975:path)  [unwired: 4 in, 2 out]
            n2996 = Unbundle(w3967) -> ()  [unwired: 3 out]
            n2997 = Strip Path(path=w3975) -> (name=w3973:string)  [unwired: 1 out]
            n2998 = Path To String(path=w3975) -> (string=w3970:string)
            "string1 3" <- w3970
            n2999 = Match Pattern(string=w3973, regular expression=".dgf") -> (before substring=→"String Control 5":string)  [unwired: 1 in, 3 out]
            n3000 = Match Pattern(string=w3970, regular expression=".dgf" ("substring (\"\")")) -> (before substring=w3980:string)  [unwired: 1 in, 3 out]
            n3001 = Concatenate Strings(w3980, ".duf" ("Substring")) -> (w3977:string)
            n3002 = String To Path(string=w3977) -> (path=w3981:path)
            n3003 = call <vilib>:"Read Characters From File.vi"("file path (dialog if empty)"=w3981, "start of read offset (chars.:0)"=60 ("start of read offset (chars.: 0)")) -> ("character string"=→"String Control 6":string)  [unwired: 4 in, 3 out]
          }
        }
        n3004 = case shown="True" "OPEN 4" {
          frame False {
          }
          frame True {
            (unwired) 0  # existing file
            w4002 = "Choose a datalog file to open"  # prompt
            n3005 = local write "OPEN 4"(FALSE ("OPEN 1")) -> ()
            n3006 = String To Path(string="C:\\LAB-IQ\\Data\\") -> (path=w3987:path)
            n3007 = File Dialog(6:"*.dgf" ("pattern"), 7:w4002, 11:w3987) -> (0:w3985:errorcluster, 3:w3993:path)  [unwired: 4 in, 2 out]
            n3008 = Unbundle(w3985) -> ()  [unwired: 3 out]
            n3009 = Strip Path(path=w3993) -> (name=w3991:string)  [unwired: 1 out]
            n3010 = Path To String(path=w3993) -> (string=w3988:string)
            "string1 4" <- w3988
            n3011 = Match Pattern(string=w3991, regular expression=".dgf") -> (before substring=→"String Control 7":string)  [unwired: 1 in, 3 out]
            n3012 = Match Pattern(string=w3988, regular expression=".dgf" ("substring (\"\")")) -> (before substring=w3998:string)  [unwired: 1 in, 3 out]
            n3013 = Concatenate Strings(w3998, ".duf" ("Substring")) -> (w3995:string)
            n3014 = String To Path(string=w3995) -> (path=w3999:path)
            n3015 = call <vilib>:"Read Characters From File.vi"("file path (dialog if empty)"=w3999, "start of read offset (chars.:0)"=60 ("start of read offset (chars.: 0)")) -> ("character string"=→"String Control 8":string)  [unwired: 4 in, 3 out]
          }
        }
      }
      frame "About" {
        # "Elapsed time\ncof\nstroke\nmean pos\nTemp\nHumidity"
        n3016 = disable-structure shown="Disabled" {
          frame Disabled {
            n3017 = case shown="True" "Export" {
              frame False {
              }
              frame True {
                w4024 = "                                      " ("string")
                w4026 = "\r"
                (unwired) i16 6 ("width (-)")
                w4103 = "\r"
                w4035 = "\r"
                n3018 = local write "Export"(FALSE ("Export")) -> ()
                n3019 = local read "String 29"() -> (w4072:string)
                n3020 = local read "String 34"() -> (w4060:string)
                n3021 = local read "String 35"() -> (w4055:string)
                n3022 = local read "String 37"() -> (w4051:string)
                n3023 = local read "String 36"() -> (w4048:string)
                n3024 = local read "String 38"() -> (w4045:string)
                n3025 = local read "String 39"() -> (w4042:string)
                n3026 = Match Pattern(string=w4072, regular expression=".dwm") -> (before substring=w4068:string)  [unwired: 1 in, 3 out]
                "before substring" <- w4068
                n3027 = local read "S 38"() -> (w4063:string)
                n3028 = local read "S 39"() -> (w4056:string)
                n3029 = local read "Temperature before test 2"() -> (w4092:dbl)
                n3030 = local read "Temperature after test 2"() -> (w4097:dbl)
                n3031 = local read "Humidity before test 2"() -> (w4078:dbl)
                n3032 = local read "Humidity after test 2"() -> (w4093:dbl)
                n3033 = local read "MWSD 2"() -> (w4089:dbl)
                n3034 = local read "WS1.4 2"() -> (w4105:dbl)
                n3035 = local read "HCF 2"() -> (w4101:dbl)
                n3036 = local read "AVP 2"() -> (w4090:dbl)
                n3037 = Concatenate Strings("1," ("string"), w4063) -> (w4062:string)
                n3038 = Concatenate Strings("2," ("string"), w4060) -> (w4059:string)
                n3039 = Concatenate Strings("3," ("string"), w4056) -> (w4058:string)
                n3040 = Concatenate Strings("4," ("string"), w4055) -> (w4054:string)
                n3041 = Concatenate Strings("5," ("string"), w4051) -> (w4052:string)
                n3042 = Concatenate Strings("6," ("string"), w4048) -> (w4049:string)
                n3043 = Concatenate Strings("7," ("string"), w4045) -> (w4046:string)
                n3044 = Concatenate Strings("8," ("string"), w4042) -> (w4043:string)
                n3045 = local read "Sample ID"() -> (w4110:string)
                n3046 = case shown="\"xlx\"" "Select File Type" {
                  tunnel: w4068 -> [w4113 w4115 w4117]
                  tunnel: [w4111 w4116 w4118] -> w4067
                  frame "xlx" {
                    n3047 = Concatenate Strings(w4113, ".xls" ("string")) -> (w4111:string)
                  }
                  frame "csv" {
                    n3048 = Concatenate Strings(w4115, ".csv" ("string")) -> (w4116:string)
                  }
                  frame "txt" {
                    n3049 = Concatenate Strings(w4117, ".txt" ("string")) -> (w4118:string)
                  }
                }
                n3050 = local read "Test Date"() -> (w4109:string)
                n3051 = local read "String 45"() -> (w4023:string)
                n3052 = local read "String 31"() -> (w4108:string)
                n3053 = local read "String 32"() -> (w4107:string)
                n3054 = local read "TITTLE"() -> (w4031:string)
                n3055 = Number To Fractional String(number=w4078, width (-)=i16 6, precision (6)=i16 2) -> (F-format string=w4077:string)  [unwired: 1 in]
                n3056 = Number To Fractional String(number=w4092, width (-)=i16 6, precision (6)=i16 2) -> (F-format string=w4098:string)  [unwired: 1 in]
                n3057 = Number To Fractional String(number=w4093, width (-)=i16 6, precision (6)=i16 2) -> (F-format string=w4091:string)  [unwired: 1 in]
                n3058 = Number To Fractional String(number=w4097, width (-)=i16 6, precision (6)=i16 2) -> (F-format string=w4096:string)  [unwired: 1 in]
                n3059 = Number To Fractional String(number=w4089, width (-)=i16 6, precision (6)=i16 2) -> (F-format string=w4087:string)  [unwired: 1 in]
                n3060 = Number To Fractional String(number=w4090, width (-)=i16 6, precision (6)=i16 2) -> (F-format string=w4088:string)  [unwired: 1 in]
                n3061 = Number To Fractional String(number=w4101, width (-)=i16 6, precision (6)=i16 2) -> (F-format string=w4102:string)  [unwired: 1 in]
                n3062 = Number To Fractional String(number=w4105, precision (6)=i16 2) -> (F-format string=w4106:string)  [unwired: 2 in]
                n3063 = local read "s.NO"() -> (w4025:string)
                n3064 = Concatenate Strings("=" ("string"), w4031) -> (w4030:string)
                n3065 = Concatenate Strings("S.No," ("string"), "                                       Parameters" ("string")) -> (w4036:string)
                n3066 = Concatenate Strings(w4103, w4062, w4077, w4103, w4059, w4098, w4103, w4058, w4091, w4103, w4054, w4096, w4103, w4052, w4087, w4103, w4049, w4088, w4103, w4046, w4102, w4103, w4043, w4106) -> (w4065:string)
                n3067 = Concatenate Strings(w4035, "," ("string"), w4023, w4025, w4024, w4107, w4110, w4024, w4108, w4109, w4035) -> (w4033:string)
                n3068 = local read "Tested by"() -> (w4039:string)
                n3069 = local read "String 33"() -> (w4040:string)
                n3070 = Concatenate Strings("," ("string"), "                                                                             " ("string")) -> (w4028:string)
                n3071 = Concatenate Strings(w4030, w4026, w4033, w4026, w4036, w4065, w4026, w4028, w4040, w4039) -> (→"export":string)
                n3072 = String To Path(string=w4067) -> (path=w4074:path)
                n3073 = local read "export"() -> (w4069:string)
                n3074 = call <vilib>:"Write Characters To File.vi"("append to file? (new file:F)"=FALSE, "character string"=w4069, "file path (dialog if empty)"=w4074) -> ()  [unwired: 2 in, 1 out]
              }
            }
          }
          frame Enabled {
          }
        }
        n3075 = case shown="True" "OK Button 17" {
          frame False {
          }
          frame True {
            (unwired) 0  # existing file
            w4327 = "Choose a datalog file to open"  # prompt
            n3076 = local write "OK Button 17"(FALSE ("OK Button 17")) -> ()
            n3077 = local read "String"() -> (w4322:string)
            n3078 = String To Path(string=w4322) -> (path=w4323:path)
            n3079 = File Dialog(6:"*.duf" ("pattern"), 7:w4327, 11:w4323) -> (0:w4314:errorcluster, 3:w4333:path)  [unwired: 4 in, 2 out]
            n3080 = Unbundle(w4314) -> ()  [unwired: 3 out]
            n3081 = Open/Create/Replace File "Open File"(file path (use dialog)=w4333) -> (refnum out=w4325:refnum<file>)  [unwired: 5 in, 2 out]
            n3082 = Strip Path(path=w4333) -> (name=w4331:string)  [unwired: 1 out]
            n3083 = Path To String(path=w4333) -> (string=w4316:string)
            n3084 = while {
              tunnel: w4325 -> [w4337]
              i -> [w4334]
              stop <- w4335 continue-if-true
              (unwired) TRUE ("line mode (F)")
              n3085 = Read from Text File "Read File"(file (use dialog)=w4337) -> (text=w4336:string)  [unwired: 3 in, 3 out]
              n3086 = local write "Numeric 16"(w4334) -> ()
              n3087 = String Length(string=w4336) -> (length=w4339:i32)
              n3088 = Greater?(x=w4339, y=1) -> (0:w4335:bool)
            }
            n3089 = local write "String 29"(w4316) -> ()
            n3090 = Search and Replace String(input string=w4316, search string=".duf", replace string=".dgf" ("replace string (\"\")")) -> (result string=→"String Indicator 4":string)  [unwired: 5 in, 3 out]
            n3091 = Match Pattern(string=w4331, regular expression=".dwm") -> (before substring=w4315:string)  [unwired: 1 in, 3 out]
            "String Indicator" <- w4315
            n3092 = Match Pattern(string=w4316, regular expression=".dwm" ("substring (\"\")")) -> (before substring=w4317:string)  [unwired: 1 in, 3 out]
            "String Indicator 3" <- w4317
            n3093 = local write "TITTLE 2"(w4315) -> ()
            n3094 = String To Path(string=w4317) -> (path=w4324:path)
            "path" <- w4324
            n3095 = call <vilib>:"Read Characters From File.vi"("file path (dialog if empty)"=w4324, "start of read offset (chars.:0)"=60 ("start of read offset (chars.: 0)")) -> ("character string"=→"String Indicator 2":string)  [unwired: 4 in, 3 out]
          }
        }
        n3096 = call <vilib>:"Query Available Printers.vi"() -> ("system configured printers"=w4016:string[])  [unwired: 9 in, 2 out]
        "System Configured Printers 2" <- w4016
        n3097 = local read "OK Button 16"() -> (w4013:bool)
        n3098 = case shown="True" "OK Button 16" {
          frame False {
          }
          frame True {
            n3099 = stacked-sequence {
              frame #0 {
                n3100 = local read "Numeric 16"() -> (w4341:i32)
                n3101 = local write "Numeric 10"(w4341) -> ()
              }
              frame #1 {
                n3102 = local read "S.NO"() -> (→"s.NO":string)
                n3103 = local read "String 29"() -> (w4345:string)
                n3104 = String To Path(string=w4345) -> (path=w4344:path)
                n3105 = Open/Create/Replace File "Open File"(file path (use dialog)=w4344) -> (refnum out=w4346:refnum<file>)  [unwired: 5 in, 2 out]
                n3106 = for {
                  N: 16 -> [_]
                  tunnel: w4346 -> [w4353]
                  i -> [w4349]
                  (unwired) TRUE ("line mode (F)")
                  n3107 = Read from Text File "Read File"(file (use dialog)=w4353) -> (text=w4347:string)  [unwired: 3 in, 3 out]
                  n3108 = Match Pattern(string=w4347, regular expression="(") -> (after substring=w4352:string)  [unwired: 1 in, 3 out]
                  n3109 = Match Pattern(string=w4352, regular expression=")") -> (before substring=w4348:string)  [unwired: 1 in, 3 out]
                  n3110 = case shown="1" w4349 {
                    tunnel: w4348 -> [w4354 w4355 _ _ w4356 w4357 w4358 w4360 w4362 w4364 w4366 w4368 w4370 w4372 _]
                    tunnel: w4347 -> [_ _ _ _ _ _ _ _ _ _ _ _ _ _ _]
                    frame 0 {
                      "TITTLE" <- w4354
                    }
                    frame 1 {
                      "Sample ID" <- w4355
                    }
                    frame 2 {
                    }
                    frame 3 {
                    }
                    frame 4 {
                      "Test Date" <- w4356
                    }
                    frame 5 {
                      "Tested by" <- w4357
                    }
                    frame 6 {
                      n3111 = Fract/Exp String To Number(string=w4358) -> (number=→"Humidity before test 2":dbl)  [unwired: 3 in, 1 out]
                    }
                    frame 7 {
                      n3112 = Fract/Exp String To Number(string=w4360) -> (number=→"Temperature before test 2":dbl)  [unwired: 3 in, 1 out]
                    }
                    frame 8 {
                      n3113 = Fract/Exp String To Number(string=w4362) -> (number=→"Humidity after test 2":dbl)  [unwired: 3 in, 1 out]
                    }
                    frame 9 {
                      n3114 = Fract/Exp String To Number(string=w4364) -> (number=→"Temperature after test 2":dbl)  [unwired: 3 in, 1 out]
                    }
                    frame 10 {
                      n3115 = Fract/Exp String To Number(string=w4366) -> (number=→"MWSD 2":dbl)  [unwired: 3 in, 1 out]
                    }
                    frame 11 {
                      n3116 = Fract/Exp String To Number(string=w4368) -> (number=→"AVP 2":dbl)  [unwired: 3 in, 1 out]
                    }
                    frame 12 {
                      n3117 = Fract/Exp String To Number(string=w4370) -> (number=→"HCF 2":dbl)  [unwired: 3 in, 1 out]
                    }
                    frame 13 {
                      n3118 = Fract/Exp String To Number(string=w4372) -> (number=→"WS1.4 2":dbl)  [unwired: 3 in, 1 out]
                    }
                    frame 14, Default {
                    }
                  }
                }
              }
              frame #2 {
              }
            }
            n3119 = local write "OK Button 16"(FALSE ("OK Button 13")) -> ()
          }
        }
        n3120 = Index Array(array=w4016, index="Select Printer 3") -> (element=w4018:string)
        "Selected Printer" <- w4018
        n3121 = case shown="True" w4013 {
          frame False {
          }
          frame True {
            n3122 = flat-sequence {
              frame #0 {
              }
              frame #1 {
                n3123 = Wait (ms)(milliseconds to wait=u32 100) -> ()  [unwired: 1 out]
              }
              frame #2 {
                n3124 = local write "OK Button 16"(FALSE ("Print 3")) -> ()
              }
            }
          }
        }
        n3125 = case shown="True" "Print" {
          tunnel: w4018 -> [_ w4310]
          frame False {
          }
          frame True {
            (unwired) i16 6 ("width (-)")
            (unwired) "TESTED BY : "
            (unwired) "TESTED DATE :"
            (unwired) "SAMPLE ID : "
            (unwired) "SAMPLE DESIGN : "
            w4268 = "\r"
            w4285 = "\r"
            # "add image"
            n3126 = local read "Sample ID"() -> (w4258:string)
            n3127 = local read "Tested by"() -> (w4261:string)
            n3128 = local read "String 34"() -> (w4248:string)
            n3129 = local read "String 45"() -> (w4228:string)
            n3130 = local read "String 35"() -> (w4243:string)
            n3131 = local read "String 37"() -> (w4241:string)
            n3132 = local read "String 32"() -> (w4263:string)
            n3133 = local read "String 36"() -> (w4238:string)
            n3134 = local read "String 31"() -> (w4262:string)
            n3135 = local read "Test Date"() -> (w4259:string)
            n3136 = local read "String 33"() -> (w4264:string)
            n3137 = local read "String 38"() -> (w4234:string)
            n3138 = local read "String 39"() -> (w4231:string)
            n3139 = local write "Print"(FALSE ("Print FF")) -> ()
            n3140 = local read "S 39"() -> (w4246:string)
